vi "ZernikeMode_Amplitude_Filter_v01.vi"(1 "Zernike Modes":i32[](array[numeric]), 2 "Zernike Mode Amp Guess Input":dbl[](array[numeric])) -> (0 "Zernike Modes Amplitudes Output":dbl[](array[numeric]))   [LabVIEW 2015]
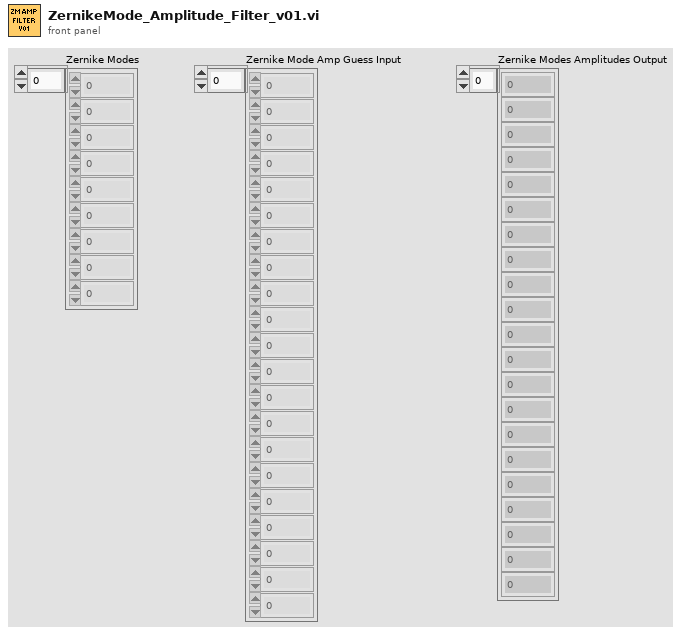
[diagram p1: front panel]
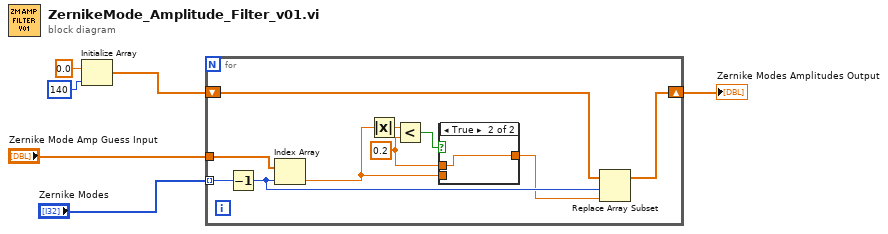
[diagram p0: block diagram]
diagram:
  n1 = Initialize Array(0.0 ("element"), 140 ("dimension size")) -> (w4:dbl[])
  n2 = for {
    tunnel: "Zernike Modes" -> [w16] mode=indexing
    tunnel: "Zernike Mode Amp Guess Input" -> [w15]
    shift-right: [w13] -> w1
    shift-left: w4 -> [w14]
    w11 = 0.2 ("y")
    n3 = Decrement(x=w16) -> (x-1=w12:i32)
    n4 = Index Array(array=w15, index=w12) -> (element=w8:dbl)
    n5 = Absolute Value(x=w8) -> (abs(x)=w10:dbl)
    n6 = Less?(x=w10, y=w11) -> (x < y?=w9:bool)
    n7 = case shown="True" w9 {
      tunnel: [w17 w18] -> w7
      tunnel: w8 -> [w17 _]
      tunnel: w11 -> [_ w18]
      frame False {
      }
      frame True {
      }
    }
    n8 = Replace Array Subset(array=w14, new element=w7, index=w12) -> (w13:dbl[])
  }
  "Zernike Modes Amplitudes Output" <- w1
